vi "Read task.vi"(8 "error in (no error)":errorcluster, 11 "DAQ  in":refnum<class "DAQ .lvclass">) -> (0 "error out":errorcluster, 2 "task":refnum<k21>, 3 "DAQ  out":refnum<class "DAQ .lvclass">)   [LabVIEW 2017, in "Hardware.lvlib" / "DAQ .lvclass"]
uses:
  DAQ .lvclass
  DAQ .lvclass/DAQ .ctl
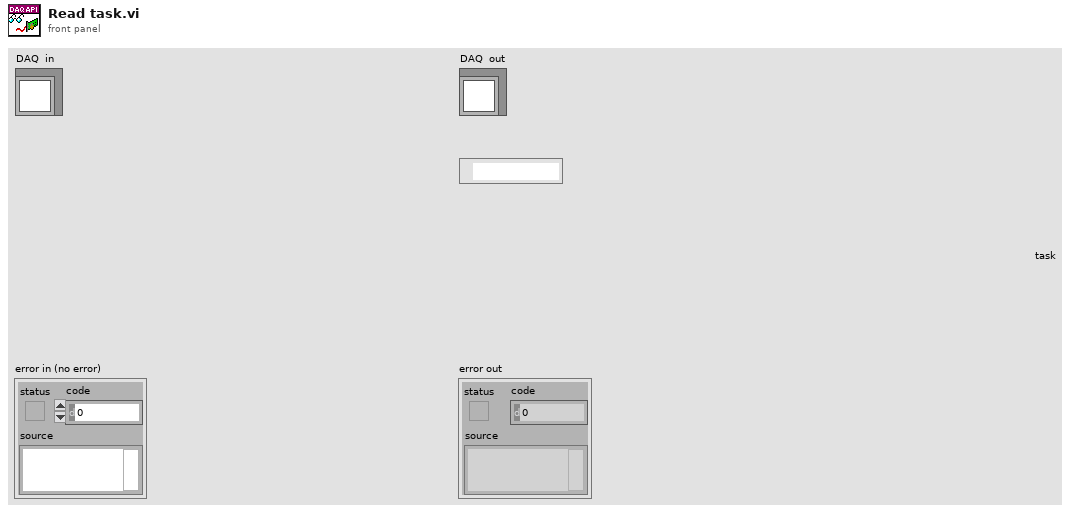
[diagram p1: front panel]
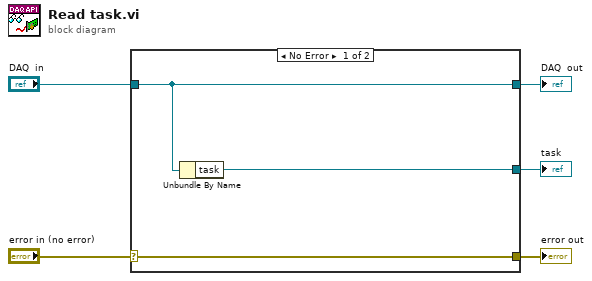
[diagram p0: block diagram]
diagram:
  n1 = case shown="No Error" "error in (no error)" {
    selector: "error in (no error)" -> [w8 w9]
    tunnel: [w8 w9] -> w4
    tunnel: [w7 w10] -> w2
    tunnel: "DAQ  in" -> [w7 w10]
    tunnel: [w6 _] -> w1
    frame No Error {
      n2 = Unbundle By Name(w7) -> ("task"=w6:refnum<k21>)
    }
    frame Error {
    }
  }
  "error out" <- w4
  "DAQ  out" <- w2
  "task" <- w1
